vi "MAIN.vi"() -> ()   [LabVIEW 2015]
uses:
  <vilib>/imath/engines/lvmath/Plug In/_Char/NIMS_CH_character datatype.ctl
  <vilib>/imath/engines/lvmath2/RunTimeEngine/Managers/WorkSpace/UID Generator.vi
  <vilib>/imath/engines/lvmath/Plug In/_Char/NIMS_CH_Character RV to String.vi
  <vilib>/imath/engines/lvmath2/RunTimeEngine/BuiltInFunctions/fopen/NIMS_fopen(Str,Enum).vi
  <vilib>/imath/engines/lvmath2/RunTimeEngine/BuiltInFunctions/size/NIMS_I32Row=size(GM).vi
  <instcachedir>/0/NIMS_I32Row=size(GM)_10ACDCB9F1F84A7E9F42C91D87611FB5.lvgen/NIMS_I32Row=size(GM)_10ACDCB9F1F84A7E9F42C91D87611FB5_000.vi
  <vilib>/imath/engines/lvmath2/RunTimeEngine/IndexRead/NIMS V(S).vi
  <instcachedir>/0/NIMS V(S)_0488751826AF41519A22953C041130DC.lvgen/NIMS V(S)_0488751826AF41519A22953C041130DC_002.vi
  <vilib>/imathl/engines/lvmath/Functions/Error Handling/Create Error.vi
  <vilib>/imath/engines/lvmath2/RunTimeEngine/RangeToken/NIMS_Range_R2 - Integer.vi
  <instcachedir>/0/NIMS_Range_R2 - Integer_396D5D4FB869421F9245109A0975AD54.lvgen/NIMS_Range_R2 - Integer_396D5D4FB869421F9245109A0975AD54_000.vi
  <vilib>/imath/engines/lvmath2/RunTimeEngine/CommandStatement/MC_CommandStatement_break.vi
  <vilib>/imath/engines/lvmath2/RunTimeEngine/IndexRead/NIMS M(S,S).vi
  <instcachedir>/0/NIMS M(S,S)_AC51E74150A542F7991B9634C66F3096.lvgen/NIMS M(S,S)_AC51E74150A542F7991B9634C66F3096_003.vi
  <vilib>/imath/engines/lvmath2/RunTimeEngine/BuiltInFunctions/fprintf/NIMS_fprintf(fid,Str,RM).vi
  <vilib>/imath/engines/lvmath2/RunTimeEngine/BuiltInFunctions/fclose/NIMS_fclose(fid).vi
  <vilib>/imath/engines/lvmath2/RunTimeEngine/Managers/SymbolTable/Clear UID.vi
  <vilib>/imath/engines/lvmath2/RunTimeEngine/ErrorHandling/NIMS_Finalize Error.vi
  <vilib>/imath/engines/lvmath2/RunTimeEngine/Managers/SymbolTable/NIMS_WorkSpace.lvlib
panel:
  out "Array 2":i32[][](array[numeric])
  in  "Path 2":path
  in  "Path":path
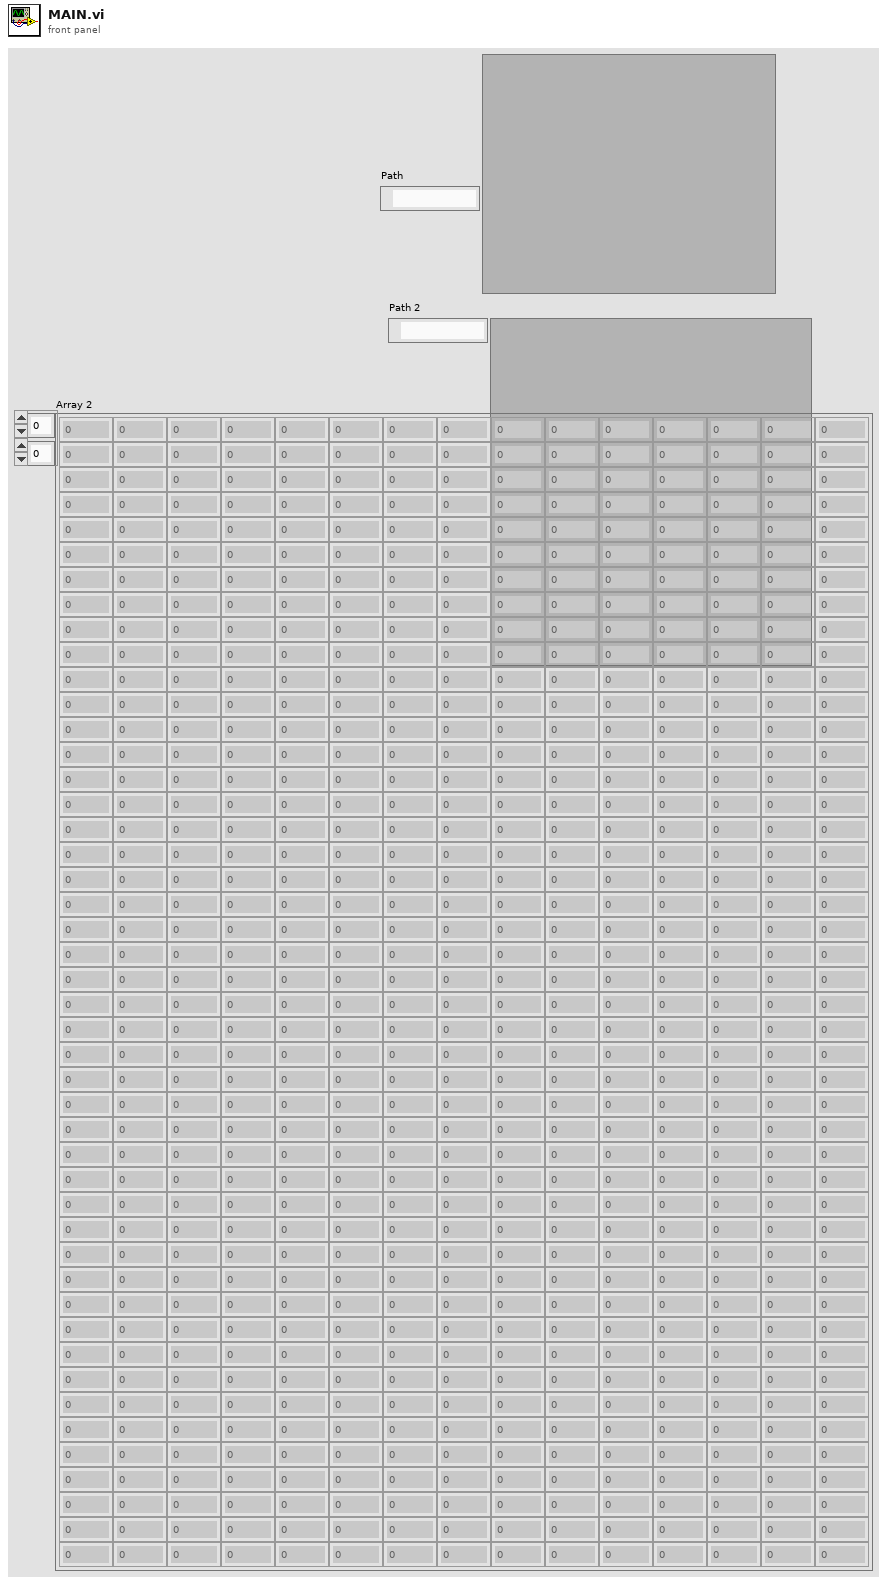
[diagram p1: front panel]
types:
  T1 = typedef "imagedata.ctl" = cluster{"image type":i32, "image depth":i32, "image":u8[], "mask":u8[], "colors":u32[], "Rectangle":cluster{"left":i16, "top":i16, "right":i16, "bottom":i16}}
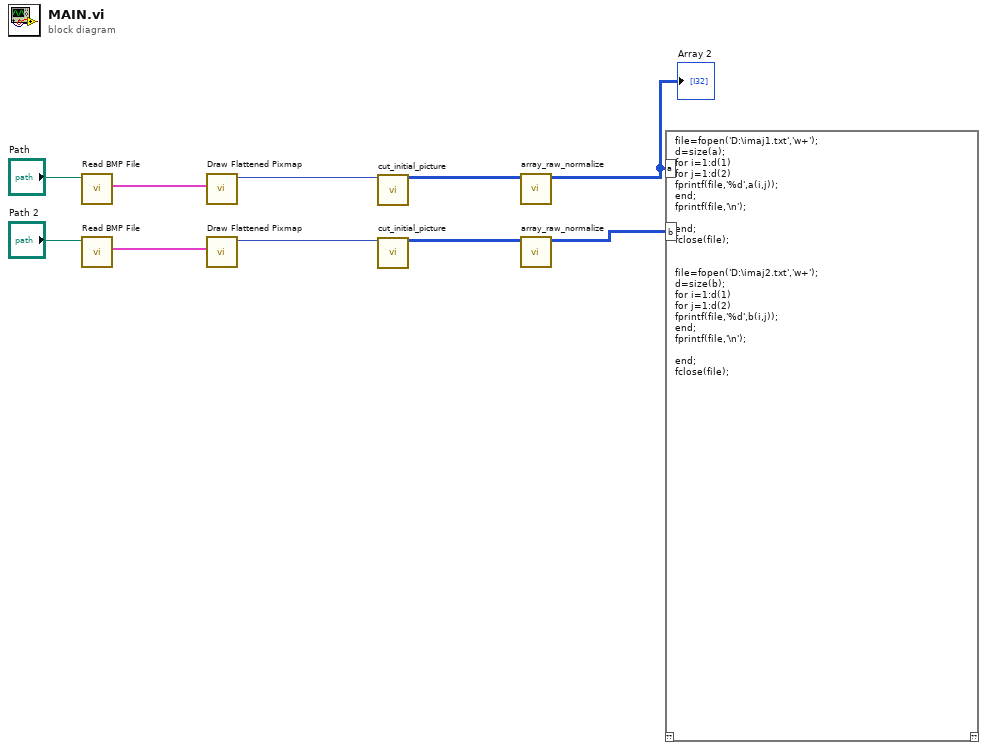
[diagram p0: block diagram]
diagram:
  n1 = call <vilib>:"Read BMP File.vi"("path to BMP file"="Path") -> ("image data"=w5:T1)  [unwired: 8 in, 2 out]
  n2 = call <vilib>:"Read BMP File.vi"("path to BMP file"="Path 2") -> ("image data"=w3:T1)  [unwired: 8 in, 2 out]
  n3 = call <vilib>:"Draw Flattened Pixmap.vi"("image data"=w5) -> ("new picture"=w9:picture)  [unwired: 8 in]
  n4 = call <vilib>:"Draw Flattened Pixmap.vi"("image data"=w3) -> ("new picture"=w10:picture)  [unwired: 8 in]
  n5 = call "cut_initial_picture.vi"("picture"=w9) -> ("new"=w8:u32[][])  [unwired: 14 in]
  n6 = call "cut_initial_picture.vi"("picture"=w10) -> ("new"=w7:u32[][])  [unwired: 14 in]
  n7 = call "array_raw_normalize.vi"("array"=w8) -> ("Array"=w2:i32[][])  [unwired: 10 in]
  "Array 2" <- w2
  n8 = call "array_raw_normalize.vi"("array"=w7) -> ("Array"=w1:i32[][])  [unwired: 10 in]
  n9 = mathscript code="file=fopen('D:\\imaj1.txt','w+');\nd=size(a);\nfor i=1:d(1)\nfor j=1:d(2)\nfprintf(file,'%d',a(i,j));\nend;\nfprintf(file,'\\n');\n\nend;\nfclose(file);\n\n\nfile=fopen('D:\\imaj2.txt','w+');\nd=size(b);\nfor i=1:d(1)\nfor j=1:d(2)\nfprintf(file,'%d',b(i,j));\nend;\nfprintf(file,'\\n');\n\nend;\nfclose(file);"("a"=w2, "b"=w1) -> ()  [unwired: 1 in, 1 out]
